vi "Flatten.vi"(8 "error in (no error)":errorcluster, 11 "Microwave Freq Scan in":refnum<class "Microwave Freq Scan.lvclass">) -> (0 "error out":errorcluster, 3 "Microwave Freq Scan out":refnum<class "Microwave Freq Scan.lvclass">)   [LabVIEW 2017, in "Microwave Freq Scan.lvclass"]
uses:
  Microwave Freq Scan.lvclass
  Microwave Freq Scan.lvclass/Microwave Freq Scan.ctl
  Global/File Locations.vi
  Scanner/Scanner.lvclass
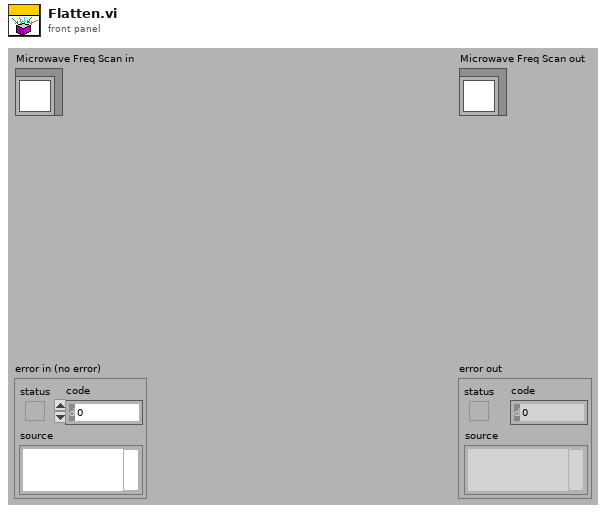
[diagram p1: front panel]
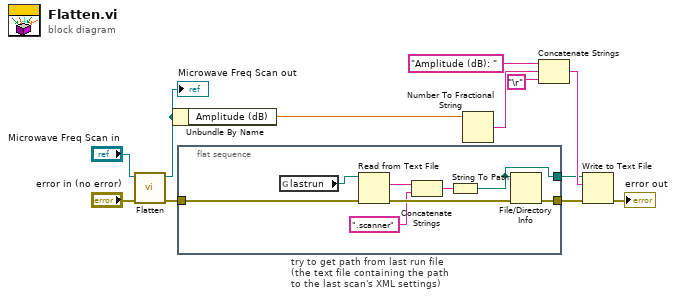
[diagram p0: block diagram]
diagram:
  n1 = call-parent "Flatten.vi"("error in (no error)"="error in (no error)", "Scanner in"="Microwave Freq Scan in") -> ("error out"=w10:errorcluster, "Scanner out"=w7:refnum<class "Microwave Freq Scan.lvclass">)  [unwired: 8 in]
  "Microwave Freq Scan out" <- w7
  n2 = Unbundle By Name(w7) -> ("Amplitude (dB)"=w6:dbl)
  n3 = flat-sequence "try to get path from last run file\n(the text file containing the path\nto the last scan's XML settings)" {
    tunnel: [w20] -> w1
    tunnel: [w17] -> w8
    tunnel: w10 -> [w16]
    frame #0 {
      n4 = global read "File Locations.vi" "lastrun"() -> (w19:path)
      n5 = Read from Text File(file (use dialog)=w19, error in=w16) -> (text=w15:string, error out=w18:errorcluster)  [unwired: 4 out]
      n6 = Concatenate Strings(w15, ".scanner") -> (w13:string)
      n7 = String To Path(string=w13) -> (path=w20:path)
      n8 = File/Directory Info(path=w20, error in=w18) -> (error out=w17:errorcluster)  [unwired: 6 out]
    }
  }
  n9 = Number To Fractional String(number=w6) -> (F-format string=w4:string)  [unwired: 3 in]
  n10 = Concatenate Strings("Amplitude (dB): ", w4, "\r") -> (w2:string)
  n11 = Write to Text File(file (use dialog)=w1, text=w2, error in=w8) -> (error out=→"error out":errorcluster)  [unwired: 1 in, 2 out]
